vi "GetGaborKernel.vi"(4 "gamma":dbl, 6 "lambd":dbl, 7 "psi":dbl=1.570796326795, 8 "error in":errorcluster, 9 "theta":dbl, 10 "sigma":dbl, 11 "ksize":T1) -> (0 "error out":errorcluster, 3 "Kernel":dbl[][](array[numeric]))   [LabVIEW 2020, in "OpenLvVision_OpenCv.lvlib"]
doc: "Returns Gabor filter coefficients."
uses:
  OpenLvVision_OpenCv.lvlib
  TypeDef/Point/2D_PointI32.ctl
  Dlls/OlvOpenCvWrapper.dll
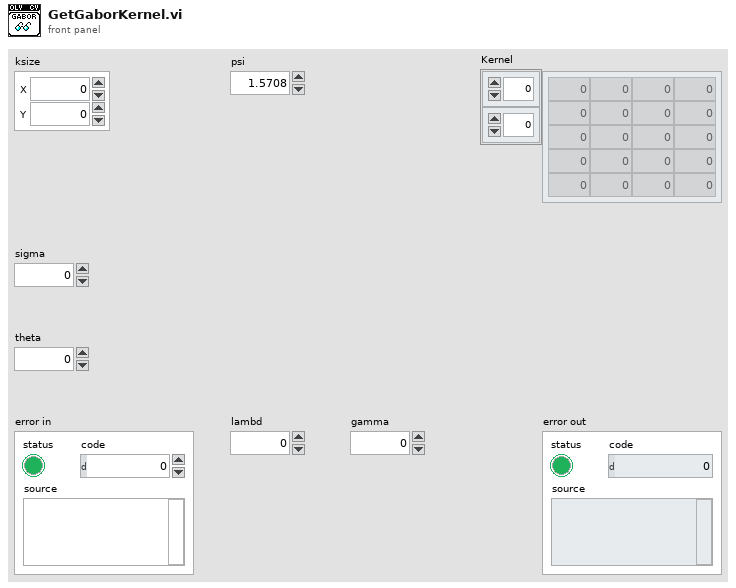
[diagram p1: front panel]
types:
  T1 = typedef "OpenLvVision_OpenCv.lvlib/2D_PointI32.ctl" = cluster{"X":i32, "Y":i32}
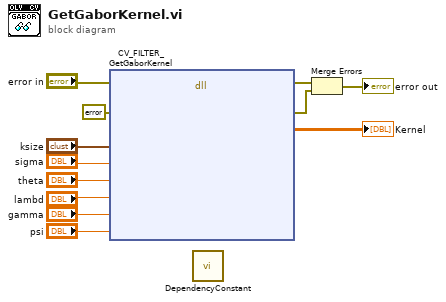
[diagram p0: block diagram]
diagram:
  n1 = dll-call lib="C:/Users/lukas/Downloads/OpenLvVision_OpenCv/SourceCode/LabView/OpenLvVision_OpenCv/Dlls/OlvOpenCvWrapper.dll" fn="CV_FILTER_GetGaborKernel"(error in="error in", "Error"=errorcluster {"status"=FALSE, "code"=0, "source"=""} ("error constant"), "kSize"="ksize", "sigma"="sigma", "theta"="theta", "lambd"="lambd", "gamma"="gamma", "psi"="psi") -> (error out=w11:errorcluster, "Error"=w10:errorcluster, "dst"=→"Kernel":dbl[][])  [unwired: 10 in, 1 out]
  n2 = call "DependencyConstant.vi"() -> ()  [unwired: 12 in]
  n3 = Merge Errors(w11, w10) -> (→"error out":errorcluster)
